vi "Core_[HSMS]Not Selected.vi"(8 "error in (no error)":errorcluster, 11 "HSMS Class in":refnum<class "HSMS Class.lvclass">) -> (0 "error out":errorcluster, 3 "HSMS Class out":refnum<class "HSMS Class.lvclass">)   [LabVIEW 2020, in "SECS Communication.lvlib" / "HSMS Class.lvclass"]
uses:
  HSMS Class.lvclass
  HSMS Class.lvclass/HSMS Class.ctl
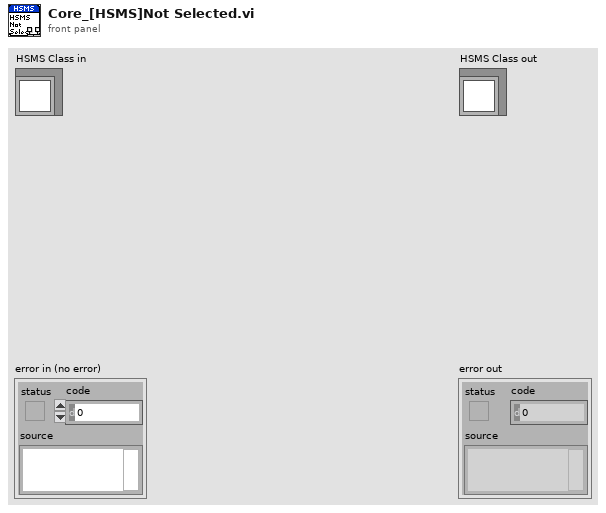
[diagram p1: front panel]
types:
  T1 = typedef "SECS Communication.lvlib/HSMS Class.lvclass/Role.ctl" = enum16{"Passive", "Active"}
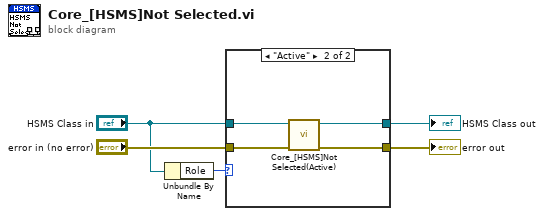
[diagram p0: block diagram]
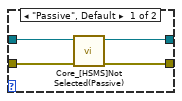
[diagram p2: hidden frame]
diagram:
  n1 = Unbundle By Name("HSMS Class in") -> ("Role"=w3:T1)
  n2 = case shown="\"Active\"" w3 {
    tunnel: "error in (no error)" -> [w9 w13]
    tunnel: "HSMS Class in" -> [w8 w12]
    tunnel: [w7 w11] -> w2
    tunnel: [w6 w10] -> w1
    frame "Passive", Default {
      n3 = call "Core_[HSMS]Not Selected(Passive).vi"("error in (no error)"=w9, "HSMS Class in"=w8) -> ("error out"=w6:errorcluster, "HSMS Class out"=w7:refnum<class "HSMS Class.lvclass">)  [unwired: 8 in]
    }
    frame "Active" {
      n4 = call "Core_[HSMS]Not Selected(Active).vi"("error in (no error)"=w13, "HSMS Class in"=w12) -> ("error out"=w10:errorcluster, "HSMS Class out"=w11:refnum<class "HSMS Class.lvclass">)  [unwired: 8 in]
    }
  }
  "error out" <- w1
  "HSMS Class out" <- w2
